vi "AddColumnAlignment.vi"(8 "error in (no error)":errorcluster, 10 "Alignment":T1, 11 "Alignment in":refnum<class "Alignment.lvclass">) -> (0 "error out":errorcluster, 3 "Alignment out":refnum<class "Alignment.lvclass">)   [LabVIEW 2021, in "LvMarkdown.lvlib" / "Alignment.lvclass"]
uses:
  Alignment.lvclass
  Alignment.lvclass/Alignment.ctl
  AlignmentEnum.ctl
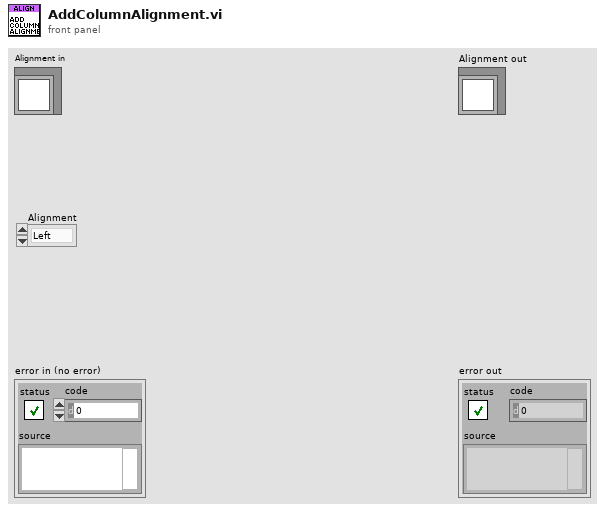
[diagram p1: front panel]
types:
  T1 = typedef "LvMarkdown.lvlib/Alignment.lvclass/AlignmentEnum.ctl" = enum16{"Left", "Center", "Right"}
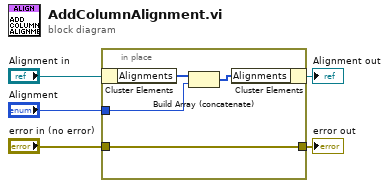
[diagram p0: block diagram]
diagram:
  n1 = in-place {
    in-place-border: "Alignment" -> [w8]
    in-place-border: "error in (no error)" -> [w6]
    in-place-border: [w6] -> w1
    n2 = in-place-cluster #1("Alignment in") -> ("Alignments"=w9:T1[])
    n3 = Build Array (concatenate)(w9, w8) -> (w7:T1[])
    n4 = in-place-cluster #1("Alignments"=w7) -> (→"Alignment out":refnum<class "Alignment.lvclass">)
  }
  "error out" <- w1
